vi "vision_webcam_V1_trigger.vi"(11 "Boolean":bool) -> ()   [LabVIEW 2017]
uses:
  <vilib>/userdefined/High Color/IMAQdx.ctl
  <vilib>/vision/Avi.llb/IMAQ AVI2 Codec Path.ctl
  Globals/Global - Configuration Options.vi
  <vilib>/vision/driver/NI_Vision_Acquisition_Software.lvlib
panel:
  out "G1 status.G1 trigger":bool
  out "Codec Names":string[](array[string])
  out "Webcam":T1(plugin-control)
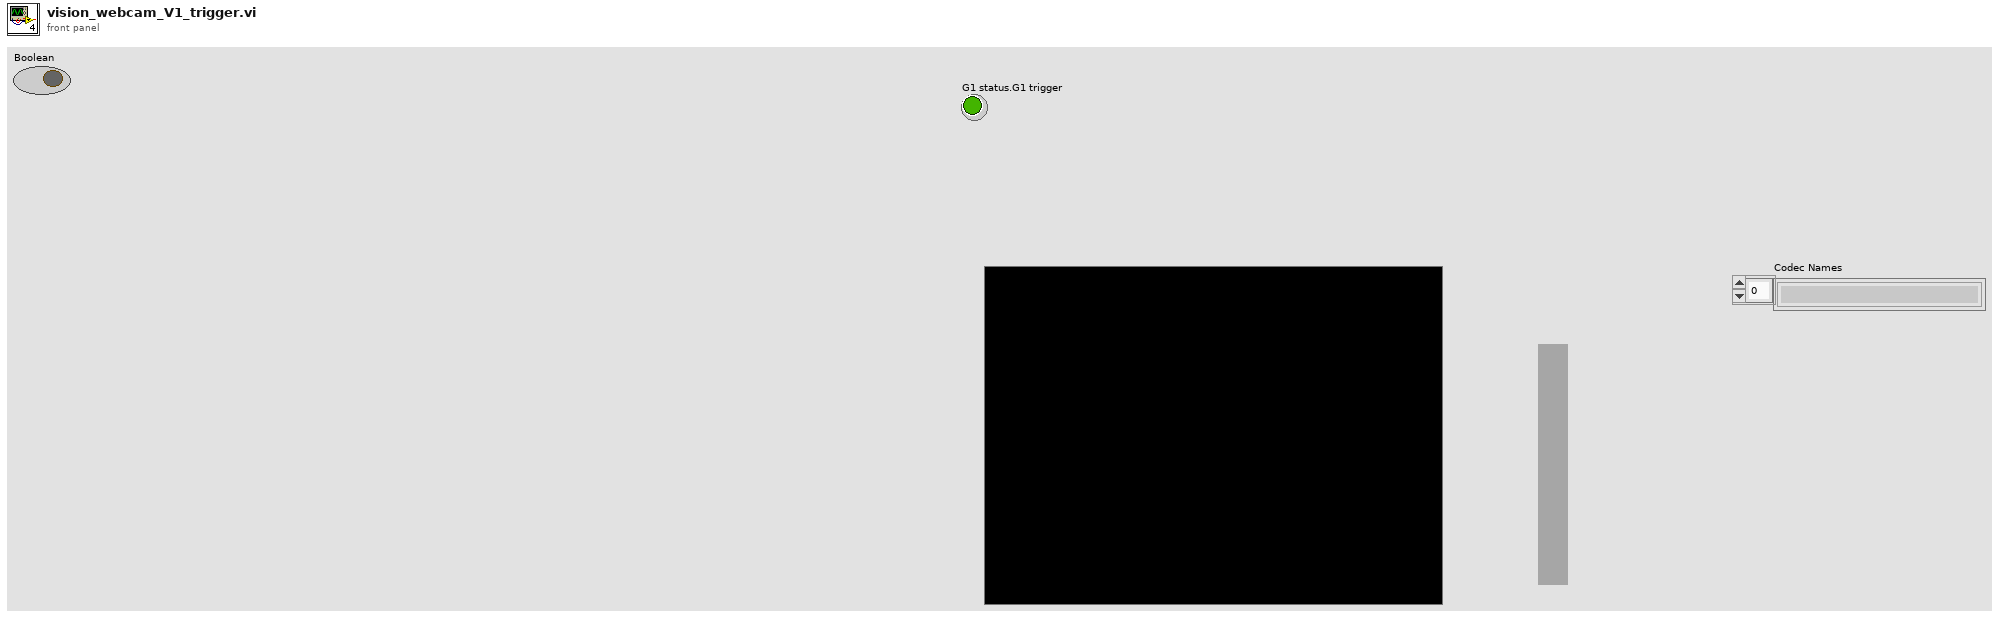
[diagram p1: front panel]
types:
  T1 = typedef "IMAQ Image.ctl" = refnum<image>
  T2 = cluster{"Tool data":cluster{"Number of teeth":sgl}, "Cutting data":cluster{"rpm":sgl}, "Limits":cluster{"Magnitude threshold":sgl, "Tolerance":sgl}, "G1 status":cluster{"G1 trigger":bool}}
  T3 = typedef "IMAQdx.ctl" = refnum<k21>
  T4 = typedef "Image Type" = u32
  T5 = typedef "IMAQ AVI2 Refnum.ctl" = refnum<k20>
  T6 = typedef "IMAQ AVI2 Codec Path.ctl" = u32
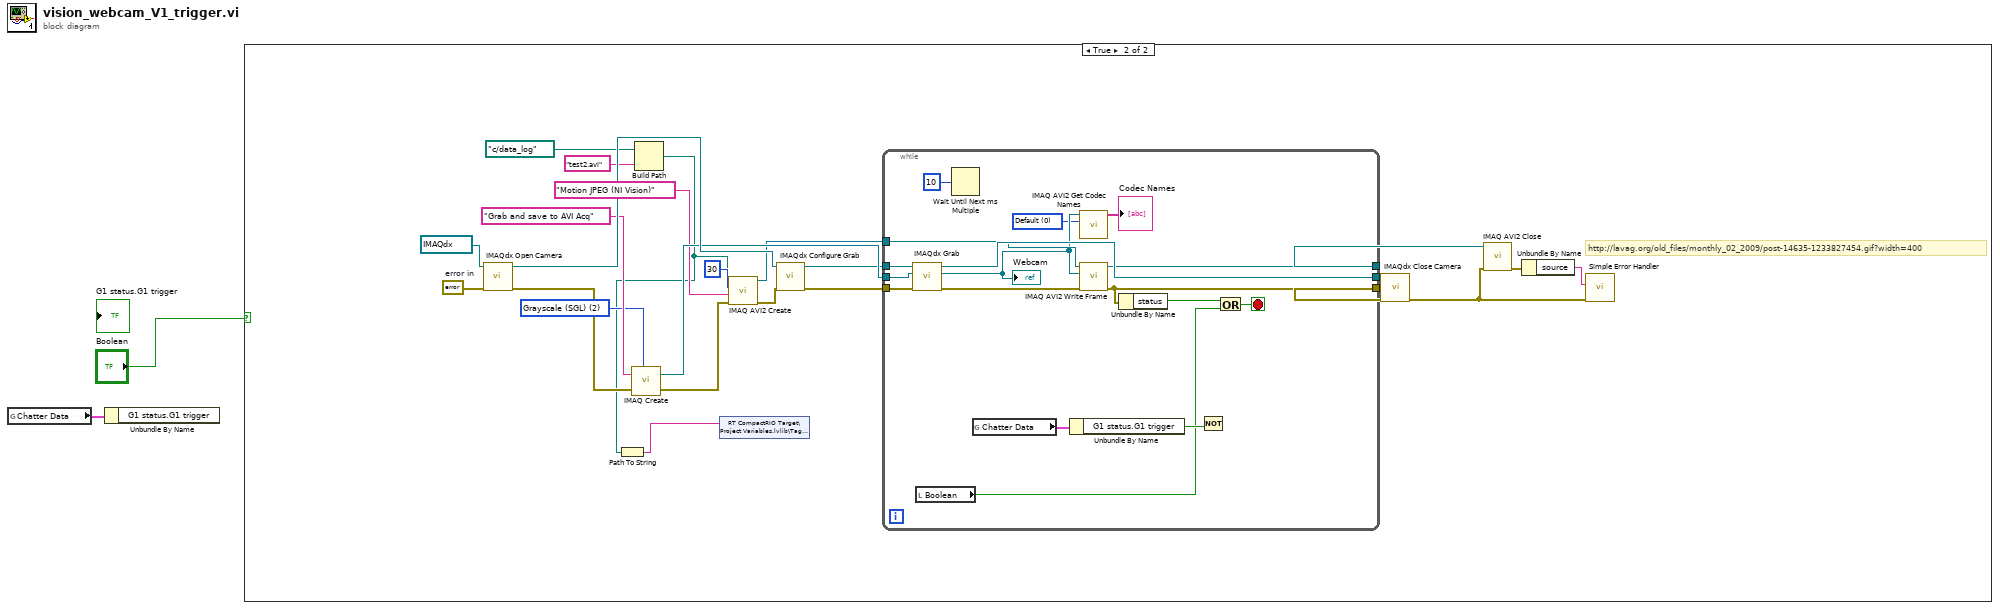
[diagram p0: block diagram]
diagram:
  n1 = global read "Global - Configuration Options.vi" "Chatter Data"() -> (w2:T2)
  n2 = Unbundle By Name(w2) -> ()  [unwired: 1 out]
  n3 = case shown="True" "Boolean" {
    frame False {
    }
    frame True {
      w10 = T4 2 items=["Grayscale (U8)", "Grayscale (I16)", "Grayscale (SGL)", "Complex (CSG)", "RGB (U32)", "HSL (U32)", "RGB (U64)", "Grayscale (U16)"] ("Image Type")
      w20 = errorcluster {"status"=FALSE, "code"=0, "source"=""}  # error in
      # "http://lavag.org/old_files/monthly_02_2009/post-14635-1233827454.gif?width=400"
      n4 = call <vilib>:"IMAQdx Open Camera.vi"("error in"=w20, "Session In"=T3 "cam0") -> ("error out"=w9:errorcluster, "Session Out"=w26:T3)  [unwired: 8 in]
      n5 = call "IMAQ Create"("Image Name"="Grab and save to AVI Acq", "Image Type"=w10, "error in (no error)"=w9) -> ("New Image"=w23:T1, "error out"=w8:errorcluster)  [unwired: 2 in]
      n6 = Build Path(base path=path "c:/data_log" ("AVI Path"), name or relative path="test2.avi") -> (appended path=w4:path)
      n7 = Path To String(path=w4) -> (string=w3:string)
      n8 = shared-variable "RT CompactRIO Target\\Project Variables.lvlib\\Tag Video"(w3) -> ()  [unwired: 1 in, 1 out]
      n9 = call "IMAQ AVI2 Create"("error in (no error)"=w8, "Codec"="Motion JPEG (NI Vision)", "Frames Per Second"=u32 30, "AVI Path"=w4) -> ("error out"=w7:errorcluster, "AVI Refnum"=w14:T5)  [unwired: 6 in]
      n10 = call <vilib>:"IMAQdx Configure Grab.vi"("error in"=w7, "Session In"=w26) -> ("error out"=w24:errorcluster, "Session Out"=w6:T3)  [unwired: 8 in]
      n11 = while {
        tunnel: w24 -> [w43]
        tunnel: w6 -> [w42]
        tunnel: w23 -> [w41]
        tunnel: [w35] -> w22
        tunnel: [w40] -> w21
        tunnel: w14 -> [w38]
        tunnel: [w37] -> w11
        stop <- w33 stop-if-true
        w31 = T6 0 items=["Default", "System", "Built in Vision"] ("Codec Source")
        n12 = call <vilib>:"IMAQdx Grab.vi"("error in"=w43, "Image In"=w41, "Session In"=w42) -> ("error out"=w36:errorcluster, "Image Out"=w32:T1, "Session Out"=w40:T3)  [unwired: 5 in, 1 out]
        "Webcam" <- w32
        n13 = local read "Boolean"() -> (w27:bool)
        n14 = Wait Until Next ms Multiple(millisecond multiple=u32 10 ("milliseconds to wait")) -> ()  [unwired: 1 out]
        n15 = global read "Global - Configuration Options.vi" "Chatter Data"() -> (w29:T2)
        n16 = Unbundle By Name(w29) -> ("G1 status.G1 trigger"=w28:bool)
        n17 = call "IMAQ AVI2 Get Codec Names"("Codec Source"=w31, "Image"=w32) -> ("Codec Names"=→"Codec Names":string[])  [unwired: 8 in, 1 out]
        n18 = call "IMAQ AVI2 Write Frame"("error in (no error)"=w36, "Image"=w32, "AVI Refnum"=w38) -> ("error out"=w35:errorcluster, "AVI Refnum (duplicate)"=w37:T5)  [unwired: 6 in, 1 out]
        n19 = Unbundle By Name(w35) -> ("status"=w34:bool)
        n20 = Not(x=w28) -> ()  [unwired: 1 out]
        n21 = Or(x=w34, y=w27) -> (x .or. y?=w33:bool)
      }
      n22 = call <vilib>:"IMAQdx Close Camera.vi"("error in"=w22, "Session In"=w21) -> ("error out"=w13:errorcluster)  [unwired: 9 in]
      n23 = call "IMAQ AVI2 Close"("error in (no error)"=w13, "AVI Refnum"=w11) -> ("error out"=w12:errorcluster)  [unwired: 9 in]
      n24 = Unbundle By Name(w12) -> ("source"=w18:string)
      n25 = call <vilib>:"Simple Error Handler.vi"("error source (\" \")"=w18, "error in (no error)"=w13) -> ()  [unwired: 3 in, 5 out]
    }
  }
